vi "Automotive ECU - Keyswitch.vi"() -> ()   [LabVIEW 2013]
doc: "Sample numeric display item."
uses:
  <vilib>/NI Veristand/Display Template Support/Display Template Support.llb/cluster_Screen Item Settings.ctl
  <vilib>/NI Veristand/Display Template Support/Display Template Support.llb/cluster_Graph Scale Settings.ctl
  <vilib>/NI Veristand/Display Template Support/Display Template Support.llb/cluster_Graph Plot Settings.ctl
  NationalInstruments.VeriStand.SystemStorage
  <vilib>/NI Veristand/Display Template Support/Display Template Support.llb/enum_Display Template Handler Minimal To Widget Msg.ctl
  <vilib>/NI Veristand/Display Template Support/Display Template Support.llb/enum_Display Template Handler Minimal To Workspace.ctl
  Support/KeySwitch Parameters.ctl
  Support/PWM Object Parameters.ctl
  <vilib>/NI Veristand/Execution/Workspace/NI VeriStand - Get Single Channel Value.vi
  <vilib>/NI Veristand/Execution/Workspace/NI_VS Workspace ExecutionAPI.lvlib
panel:
  in  "Knob":u8(knob) max=100 step=1 scale=0.0..4.0
  in  "NIVS.System Definition Root":refnum<k24>
  in  "NIVS.Gateway IP Address":string
  out "Label":string="Numeric"
  in  "Item.Data":T1
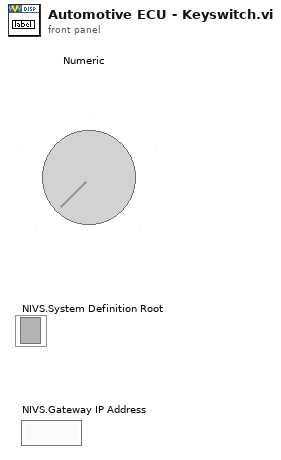
[diagram p1: front panel]
types:
  T1 = typedef "cluster_Screen Item Settings.ctl" = cluster{"Template VI":string, "Position X":i32, "Position Y":i32, "Custom":string, "Show Title Bar":bool, "ID":i32, "Always On Top":bool, "Allow Resize":bool, "Allow Minimize":bool, "Allow Close":bool, "Size to Screen":bool, "Screen.ID":i32, "State":enum16{"Normal", "New"}, "Title":string, "Window Bounds":cluster{"[0]":i16, "[1]":i16, "[2]":i16, "[3]":i16}, "Channel Ref":u64, "Unit":string, "Default Units?":bool, "Flash Limit?":bool, "Color 1":u32, "Color 2":u32, "Color 3":u32, "Color 4":u32, "Bck Color":u32, "Fore Color":u32, "Limit 1":dbl, "Limit 2":dbl, "Limit 3":dbl, "Limit 4":dbl, "Limit Mode 1":i32, "Limit Mode 2":i32, "Limit Mode 3":i32, "Limit Mode 4":i32, "Scale Precision":i32, "Scale Min":dbl, "Scale Max":dbl, "Format":i32, "Precision":i32, "Background Type":i32, "IDs":i32[], "Units":string[], "Labels":string[], "Scale Factor":dbl, "Scale Offset":dbl, "YScale Index":u32[], "XScale":T2, "YScales":T2[], "Plots":T3[], "Update Period":dbl, "History Length":dbl, "My.Ref":refnum<vi>, "Is Control?":bool, "Channel Paths":string[], "Custom Data":variant}
  T2 = typedef "cluster_Graph Scale Settings.ctl" = cluster{"Format":u8, "Precision":u8, "Fit":u8, "Label":string, "Use Default Label":bool, "Label Visible":bool, "Min":dbl, "Max":dbl}
  T3 = typedef "cluster_Graph Plot Settings.ctl" = cluster{"Bar Style":u8, "Fill To":i16, "Fill/PtColor":u32, "Line Style":u8, "Line Width":u8, "Color":u32, "Interp":u8, "Point Style":u8}
  T4 = typedef "enum_Display Template Handler Minimal To Workspace.ctl" = cluster{"Operation":enum16{"SetCustomData", "DeleteItem"}, "Data":variant}
  T5 = typedef "enum_Display Template Handler Minimal To Widget Msg.ctl" = enum16{"Stop", "LaunchConfigDialog"}
  T6 = typedef "KeySwitch Parameters.ctl" = cluster{"PWM Config":T7, "PWM Output Settings":dbl[], "BG color":u32, "Obj Color":u32, "Initialized?":bool, "# Positions":u8, "Display Strings":string[], "Default Control Values":variant[]}
  T7 = typedef "PWM Object Parameters.ctl" = cluster{"RIO?":bool, "Label":string, "PWM Channel Path":cluster{"NodePathArray":string[], "Node Path":string}}
  T8 = typedef "NI_VS Workspace ExecutionAPI.lvlib/WorkspaceAPI.ctl" = refnum<k24>
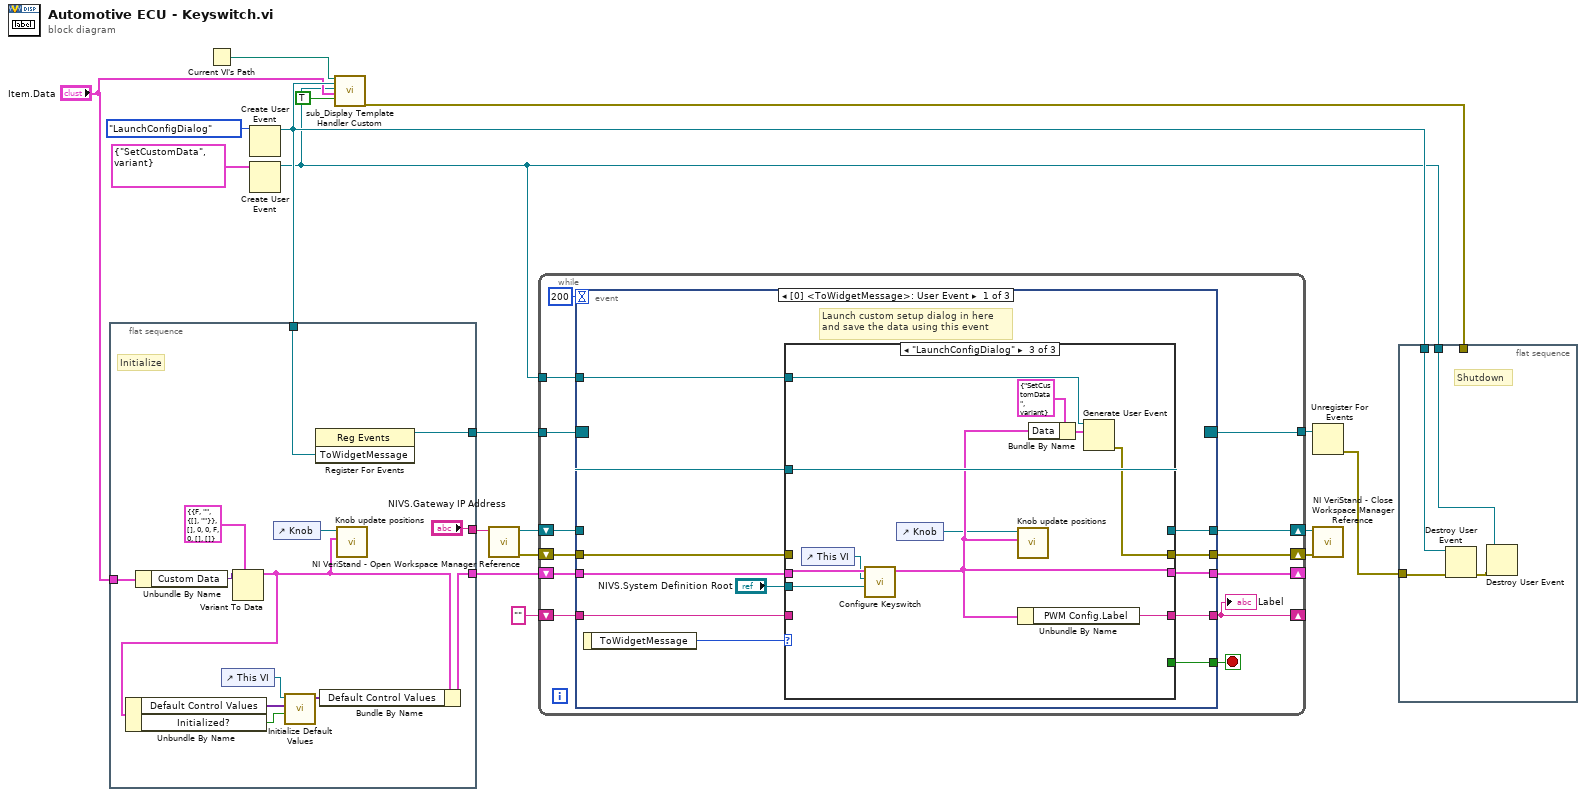
[diagram p0: block diagram]
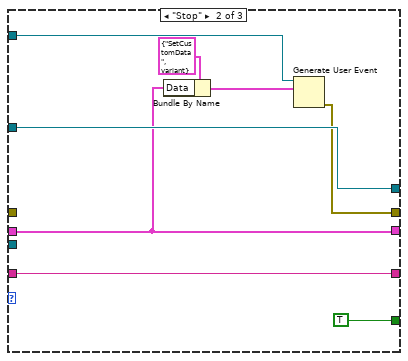
[diagram p3: hidden frame]
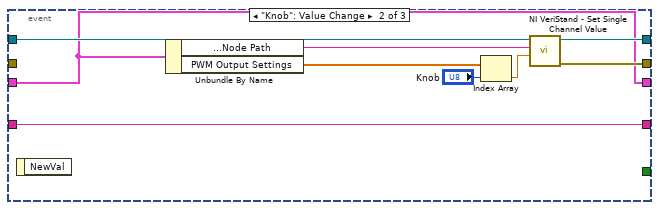
[diagram p4: hidden frame]
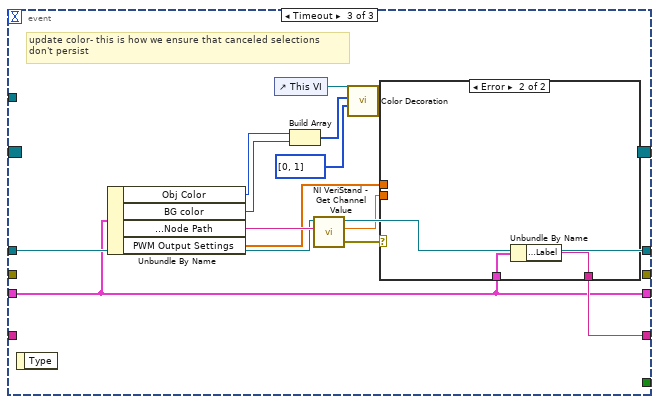
[diagram p5: hidden frame]
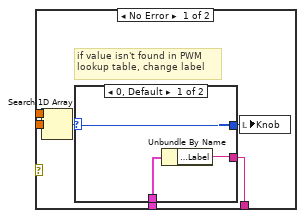
[diagram p6: hidden frame]
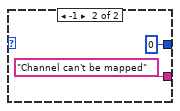
[diagram p7: hidden frame]
diagram:
  n1 = flat-sequence {
    tunnel: [w31] -> w16
    tunnel: w13 -> [w30]
    tunnel: "Item.Data" -> [w29]
    tunnel: [w19] -> w7
    tunnel: ["NIVS.Gateway IP Address"] -> w2
    frame #0 {
      # "Initialize"
      n2 = Unbundle By Name(w29) -> ("Custom Data"=w28:variant)
      n3 = control-ref of="This VI"() -> (w22:refnum<vi>)
      n4 = Variant To Data(type=T6 {"PWM Config"={"RIO?"=FALSE, "Label"="", "PWM Channel Path"={"NodePathArray"=[], "Node Path"=""}}, "PWM Output Settings"=[], "BG color"=0, "Obj Color"=0, "Initialized?"=FALSE, "# Positions"=0, "Display Strings"=[], "Default Control Values"=[]} ("Cluster"), Variant=w28) -> (data=w20:T6)  [unwired: 1 in, 1 out]
      n5 = Unbundle By Name(w20) -> ("Default Control Values"=w23:variant[], "Initialized?"=w21:bool)
      n6 = control-ref of="Knob"() -> (w25:refnum<vi>)
      n7 = call "Initialize Default Values.vi"("Initialized?"=w21, "Default Control Values in"=w23, "VI in"=w22) -> ("Default Control Values out"=w24:variant[])  [unwired: 7 in, 1 out]
      n8 = register-events(w30) -> (reference out=w31:refnum<event-registration>)  [unwired: 2 in, 1 out]
      n9 = Bundle By Name(cluster=w20, "Default Control Values"=w24) -> (w19:T6)
      n10 = call "Knob update positions.vi"("Keyswitch Cluster"=w20, "Knob refference  in"=w25) -> ()  [unwired: 9 in, 1 out]
    }
  }
  n11 = Current VI's Path() -> (path=w11:path)
  n12 = Create User Event(user event datatype=enum_Display_Template_Handler_Minimal_To_Widget_Msg."LaunchConfigDialog" ("ToWidgetMessage")) -> (user event=w13:refnum<user-event>)  [unwired: 1 in, 1 out]
  n13 = Create User Event(user event datatype=T4 {"Operation"=enum."SetCustomData", "Data"=variant} ("Data")) -> (user event=w9:refnum<user-event>)  [unwired: 1 in, 1 out]
  n14 = call <vilib>:"sub_Display Template Handler Custom.vi"("Parent.Path"=w11, "ToWidgetEvent"=w13, "ToWorkspace"=w9, "Item.Data"="Item.Data", "Resizable"=TRUE) -> ("error out"=w18:errorcluster)  [unwired: 14 in]
  n15 = call <vilib>:"NI VeriStand - Open Workspace Manager Reference.vi"("Gateway IP Address (\"\": localhost)"=w2) -> ("error out"=w5:errorcluster, "WorkspaceManager"=w6:T8)  [unwired: 9 in]
  n16 = while {
    tunnel: w16 -> [w44]
    tunnel: [w42] -> w15
    tunnel: w9 -> [w41]
    shift-right: [w34] -> _
    shift-left: w7 -> [w40]
    shift-right: [w37] -> w4
    shift-left: w6 -> [w39]
    shift-right: [w35] -> w3
    shift-left: w5 -> [w38]
    shift-right: [w32] -> _
    shift-left: "" ("Out") -> [w36]
    stop <- w43 stop-if-true
    n17 = event shown="[0] <ToWidgetMessage>: User Event" {
      selector: w44 -> [_ _ _]
      dyn-events: [_ _ _] -> w42
      timeout: 200 -> [_ _ _]
      tunnel: [w55 _ _] -> w43
      tunnel: w41 -> [w54 _ _]
      tunnel: w40 -> [w50 w82 w90]
      tunnel: w39 -> [w53 w88 w95]
      tunnel: w38 -> [w48 _ _]
      tunnel: [w52 w84 w94] -> w37
      tunnel: [w47 w85 _] -> w35
      tunnel: [w46 w83 w91] -> w32
      tunnel: w36 -> [w45 w83 _]
      tunnel: [w49 w82 w90] -> w34
      event User Event {
        # "Launch custom setup dialog in here\nand save the data using this event"
        n18 = event-data() -> ("ToWidgetMessage"=w56:T5)  [unwired: 1 out]
        n19 = case shown="\"LaunchConfigDialog\"" w56 {
          tunnel: [_ TRUE _] -> w55
          tunnel: w54 -> [_ w64 w74]
          tunnel: w53 -> [w60 w67 w79]
          tunnel: [w60 w67 w79] -> w52
          tunnel: "NIVS.System Definition Root" -> [_ _ w77]
          tunnel: w50 -> [w59 w63 w78]
          tunnel: [w59 w63 w70] -> w49
          tunnel: w48 -> [w57 _ _]
          tunnel: [w57 w62 w73] -> w47
          tunnel: [w58 w61 w72] -> w46
          tunnel: w45 -> [w58 w61 _]
          frame Default {
          }
          frame "Stop" {
            n20 = Bundle By Name(cluster=T4 {"Operation"=enum."SetCustomData", "Data"=variant} ("event data"), "Data"=w63) -> (w65:T4)
            n21 = Generate User Event(user event=w64, event data cluster=w65) -> (error out=w62:errorcluster)  [unwired: 2 in, 1 out]
          }
          frame "LaunchConfigDialog" {
            n22 = control-ref of="This VI"() -> (w71:refnum<vi>)
            n23 = call "Configure Keyswitch.vi"("NIVS.System Definition Root"=w77, "VI Reference"=w71, "FNR Data in"=w78) -> ("FNR Data Out"=w70:T6)  [unwired: 7 in, 1 out]
            n24 = control-ref of="Knob"() -> (w69:refnum<vi>)
            n25 = call "Knob update positions.vi"("Keyswitch Cluster"=w70, "Knob refference  in"=w69) -> ()  [unwired: 9 in, 1 out]
            n26 = Unbundle By Name(w70) -> ("PWM Config.Label"=w72:string)
            n27 = Bundle By Name(cluster=T4 {"Operation"=enum."SetCustomData", "Data"=variant} ("event data"), "Data"=w70) -> (w76:T4)
            n28 = Generate User Event(user event=w74, event data cluster=w76) -> (error out=w73:errorcluster)  [unwired: 2 in, 1 out]
          }
        }
      }
      event "Knob": Value Change {
        n29 = event-data() -> ()  [unwired: 2 out]
        n30 = Unbundle By Name(w82) -> ("PWM Config.PWM Channel Path.Node Path"=w87:string, "PWM Output Settings"=w80:dbl[])
        n31 = Index Array(array=w80, index="Knob") -> (element=w86:dbl)
        n32 = call <vilib>:"NI VeriStand - Set Single Channel Value.vi"("Value"=w86, "Channel"=w87, "WorkspaceManager in"=w88) -> ("error out"=w85:errorcluster, "WorkspaceManager out"=w84:T8)  [unwired: 7 in]
      }
      event Timeout {
        # "update color- this is how we ensure that canceled selections \ndon't persist"
        n33 = event-data() -> ()  [unwired: 2 out]
        n34 = Unbundle By Name(w90) -> ("Obj Color"=w98:u32, "BG color"=w97:u32, "PWM Config.PWM Channel Path.Node Path"=w96:string, "PWM Output Settings"=w93:dbl[])
        n35 = control-ref of="This VI"() -> (w101:refnum<vi>)
        n36 = Build Array(w98, w97) -> (w99:u32[])
        n37 = call-poly <vilib>:"NI VeriStand - Get Channel Value.vi"("Channel"=w96, "WorkspaceManager in"=w95) -> ("error out"=w89:errorcluster, "Value"=w92:dbl, "WorkspaceManager out"=w94:T8)  [unwired: 7 in]
        n38 = call "Color Decoration.vi"("VI reference"=w101, "Color Array"=w99, "Index Array"=u32[] [0, 1]) -> ()  [unwired: 7 in, 1 out]
        n39 = case shown="Error" w89 {
          tunnel: w93 -> [w107 _]
          tunnel: w92 -> [w106 _]
          tunnel: [w103 w113] -> w91
          tunnel: w90 -> [w102 w114]
          frame No Error {
            # "if value isn't found in PWM\nlookup table, change label"
            n40 = Search 1D Array(1D array=w107, element=w106) -> (index of element=w105:i32)  [unwired: 1 in]
            n41 = case shown="0, Default" w105 {
              selector: w105 -> [w110 _]
              tunnel: [w110 0 ("index of element")] -> w104
              tunnel: [w109 "Channel can't be mapped" ("Out")] -> w103
              tunnel: w102 -> [w108 _]
              frame 0, Default {
                n42 = Unbundle By Name(w108) -> ("PWM Config.Label"=w109:string)
              }
              frame -1 {
              }
            }
            n43 = local write "Knob"(w104) -> ()
          }
          frame Error {
            n44 = Unbundle By Name(w114) -> ("PWM Config.Label"=w113:string)
          }
        }
      }
    }
    "Label" <- w32
  }
  n45 = Unregister For Events(event registration refnum=w15) -> (error out=w14:errorcluster)  [unwired: 1 in]
  n46 = call <vilib>:"NI VeriStand - Close Workspace Manager Reference.vi"("error in (no error)"=w3, "WorkspaceManager"=w4) -> ()  [unwired: 9 in, 1 out]
  n47 = flat-sequence {
    tunnel: w18 -> [_]
    tunnel: w14 -> [w117]
    tunnel: w13 -> [w118]
    tunnel: w9 -> [w115]
    frame #0 {
      # "Shutdown"
      n48 = Destroy User Event(user event=w118, error in=w117) -> (error out=w116:errorcluster)
      n49 = Destroy User Event(user event=w115, error in=w116) -> ()  [unwired: 1 out]
    }
  }
